vi "example.vi"() -> ()   [LabVIEW 2022 SP3]
uses:
  cfitsio-bitpix.ctl
  gfitsio-write-image-subset-i32-2d.vi
  gfitsio-read-image-subset-i32-2d.vi
  <vilib>/picture/picture.llb/Draw True-Color Pixmap.vi
  gfitsio.lvlib
panel:
  in  "Tab Control":enum32{"Complete Image", "Red", "Green", "Blue"}(tab)
  out "Complete Image":picture
  out "Red":picture
  out "Green":picture
  out "Blue":picture
  # "Run the VI to create a FITS file from a BMP image stored on disk and then read back the FITS file to populate the image below."
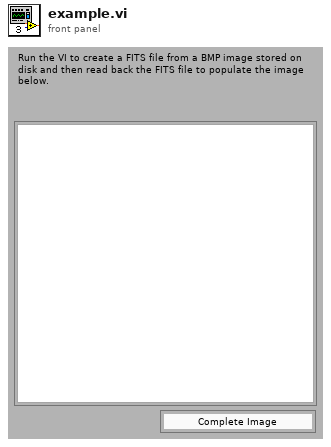
[diagram p1: front panel]
types:
  T1 = enum16{"open", "open or create", "create", "create or replace"}
  T2 = enum16{"open", "open or create", "create or replace", "create", "open (read only)"}
  T3 = typedef "gfitsio.lvlib/cfitsio-bitpix.ctl" = i32
  T4 = typedef "imagedata.ctl" = cluster{"image type":i32, "image depth":i32, "image":u8[], "mask":u8[], "colors":u32[], "Rectangle":cluster{"left":i16, "top":i16, "right":i16, "bottom":i16}}
  T5 = typedef "gfitsio.lvlib/gfitsio-refnum.ctl" = refnum<k1>
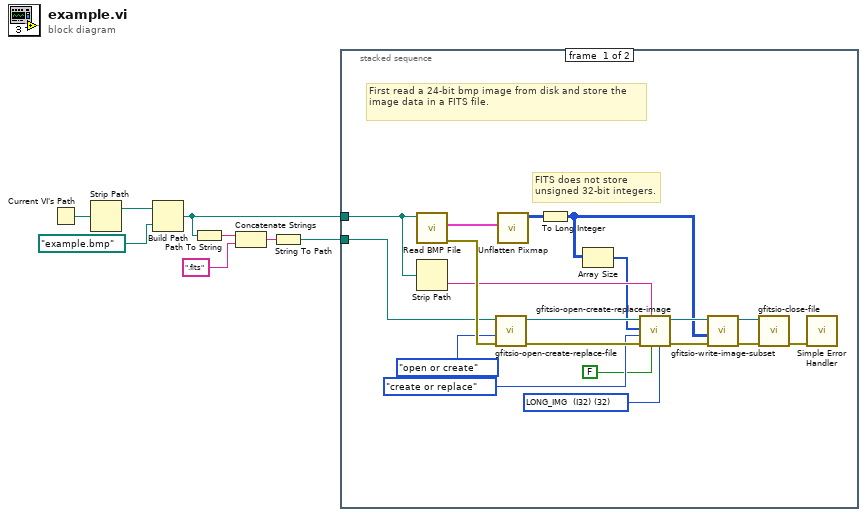
[diagram p0: block diagram]
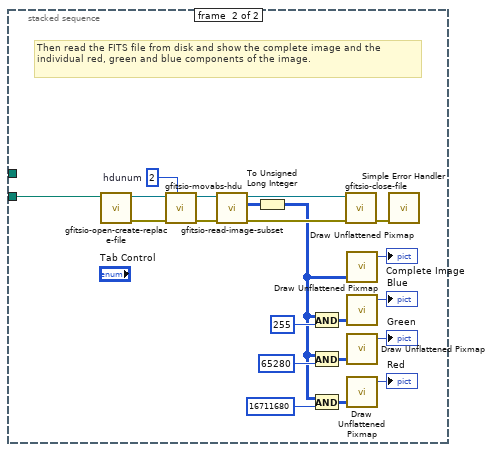
[diagram p2: hidden frame]
diagram:
  n1 = Current VI's Path() -> (path=w6:path)
  n2 = Strip Path(path=w6) -> (stripped path=w7:path)  [unwired: 1 out]
  n3 = Build Path(base path=w7, name or relative path=path "example.bmp" ("path to BMP file")) -> (appended path=w2:path)
  n4 = Path To String(path=w2) -> (string=w3:string)
  n5 = Concatenate Strings(w3, ".fits" ("string")) -> (w5:string)
  n6 = String To Path(string=w5) -> (path=w1:path)
  n7 = stacked-sequence {
    tunnel: w2 -> [w9 _]
    tunnel: w1 -> [w10 w28]
    frame #0 {
      w14 = T3 32 items=["<invalid type>"=0, "BYTE_IMG  (U8)"=8, "SHORT_IMG  (I16)"=16, "USHORT_IMG  (U16)"=20, "LONG_IMG  (I32)"=32, "ULONG_IMG  (U32)"=40, "FLOAT_IMG  (SGL)"=-32, "DOUBLE_IMG  (DBL)"=-64] ("image data type")
      # "First read a 24-bit bmp image from disk and store the image data in a FITS file."
      # "FITS does not store unsigned 32-bit integers."
      n8 = call <vilib>:"Read BMP File.vi"("path to BMP file"=w9) -> ("error out"=w21:errorcluster, "image data"=w13:T4)  [unwired: 8 in, 1 out]
      n9 = Strip Path(path=w9) -> (name=w17:string)  [unwired: 1 out]
      n10 = call "gfitsio-open-create-replace-file.vi"("error in (no error)"=w21, "function (open)"=T2."open or create", "file path (dialog if empty)"=w10) -> ("error out"=w26:errorcluster, "gfits refnum"=w27:T5)  [unwired: 6 in, 1 out]
      n11 = call <vilib>:"Unflatten Pixmap.vi"("image data"=w13) -> ("24-bit pixmap"=w20:u32[][])  [unwired: 4 in, 6 out]
      n12 = To Long Integer(number=w20) -> (32bit integer=w16:i32[][])
      n13 = Array Size(array=w16) -> (size(s)=w15:i32[])
      n14 = call "gfitsio-open-create-replace-image.vi"("image data type"=w14, "advisory dialog? (display:T)"=FALSE, "hdu name (dialog if empty)"=w17, "error in (no error)"=w26, "function (create or replace)"=T1."create or replace" ("function (open or create)"), "naxes"=w15, "gfits refnum"=w27) -> ("error out"=w25:errorcluster, "dup gfits refnum"=w22:T5)  [unwired: 2 in, 1 out]
      n15 = call-poly "gfitsio-write-image-subset.vi"("error in (no error)"=w25, "data"=w16, "gfits refnum"=w22) -> ("error out"=w24:errorcluster, "dup gfits refnum"=w23:T5)  [unwired: 7 in]
      n16 = call "gfitsio-close-file.vi"("error in (no error)"=w24, "gfits refnum"=w23) -> ("error out"=w12:errorcluster)  [unwired: 8 in, 1 out]
      n17 = call <vilib>:"Simple Error Handler.vi"("error in (no error)"=w12) -> ()  [unwired: 4 in, 5 out]
    }
    frame #1 {
      w41 = 2  # hdunum
      # "Then read the FITS file from disk and show the complete image and the individual red, green and blue components of the image."
      n18 = call "gfitsio-open-create-replace-file.vi"("file path (dialog if empty)"=w28) -> ("error out"=w48:errorcluster, "gfits refnum"=w47:T5)  [unwired: 8 in, 1 out]
      n19 = call "gfitsio-movabs-hdu.vi"("hdunum"=w41, "error in (no error)"=w48, "gfits refnum"=w47) -> ("error out"=w46:errorcluster, "dup gfits refnum"=w45:T5)  [unwired: 6 in, 1 out]
      n20 = call-poly "gfitsio-read-image-subset.vi"("error in (no error)"=w46, "gfits refnum"=w45) -> ("error out"=w44:errorcluster, "data"=w40:i32[][], "dup gfits refnum"=w43:T5)  [unwired: 7 in]
      n21 = To Unsigned Long Integer(number=w40) -> (unsigned 32bit integer=w29:u32[][])
      n22 = And(x=w29, y=u32 255) -> (x .and. y?=w36:u32[][])
      n23 = And(x=w29, y=u32 65280) -> (x .and. y?=w33:u32[][])
      n24 = And(x=w29, y=u32 16711680) -> (x .and. y?=w31:u32[][])
      n25 = call "gfitsio-close-file.vi"("error in (no error)"=w44, "gfits refnum"=w43) -> ("error out"=w42:errorcluster)  [unwired: 8 in, 1 out]
      n26 = call-poly <vilib>:"Draw Unflattened Pixmap.vi"("data (RGB format)"=w29) -> ("new picture"=→"Complete Image":picture)  [unwired: 8 in]
      n27 = call-poly <vilib>:"Draw Unflattened Pixmap.vi"("data (RGB format)"=w36) -> ("new picture"=→"Blue":picture)  [unwired: 8 in]
      n28 = call-poly <vilib>:"Draw Unflattened Pixmap.vi"("data (RGB format)"=w33) -> ("new picture"=→"Green":picture)  [unwired: 8 in]
      n29 = call-poly <vilib>:"Draw Unflattened Pixmap.vi"("data (RGB format)"=w31) -> ("new picture"=→"Red":picture)  [unwired: 8 in]
      n30 = call <vilib>:"Simple Error Handler.vi"("error in (no error)"=w42) -> ()  [unwired: 4 in, 5 out]
    }
  }
